vi "CambiaSignoString.vi"(1 "result":string[](array[string])) -> (0 "result out":dbl[](array[numeric]) format="%.1g")   [LabVIEW 2019, in "Prueba04.lvclass"]
doc: "Cambia el punto decimal de un string desde \"punto\" a \"coma\" y lo vuelve a string"
uses:
  Prueba04.lvclass
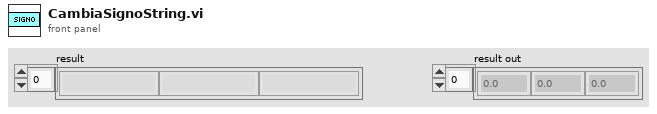
[diagram p1: front panel]
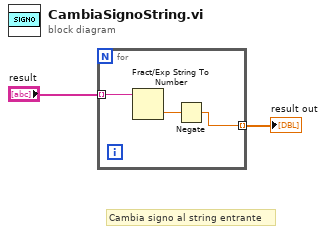
[diagram p0: block diagram]
diagram:
  # "Cambia signo al string entrante"
  n1 = for {
    tunnel: "result" -> [w5] mode=indexing
    tunnel: [w3] -> w1 mode=indexing
    n2 = Fract/Exp String To Number(string=w5) -> (number=w4:dbl)  [unwired: 3 in, 1 out]
    n3 = Negate(x=w4) -> (-x=w3:dbl)
  }
  "result out" <- w1
